vi "Action Worker Mode Example.vi"() -> ()   [LabVIEW 2017, in "Action Worker Mode Example.lvlib"]
doc: "### Caller Program (Action Worker Mode Example.vi)\n\n#### Overview\n\nDemonstrates the Worker Mode within the CSM framework. In this example, four workers run in the background, collectively forming a CSM module in Worker Mode.\n\n#### Introduction\n\nThis example demonstrates the Worker Mode within the CSM framework. In Worker Mode, multiple cloneable CSM instances run as nodes. To avoid naming conflicts, the module name is appended with a \"#\" suffix, informing the CSM framework that this is a worker module. When a message is sent to the workers, the message is handled using a fair queuing mechanism, where the first available worker module processes the message. From an external perspective, the system behaves as if only a single module is running, and all CSM concepts, such as synchronous, asynchronous, and broadcast, remain unchanged.\n\nIn this example, four workers run in the background.\n\n#### Steps\n\n- Step1: Use the Advanced VI to mark the CSM module as Worker Mode (adding `#` as a suffix). If you are familiar with CSM rules, you can also type the correct name suffix directly without using this VI. Then, asynchronously call the 4 worker CSM modules without waiting for a reply. Alternatively, you can call the 4 worker CSM modules synchronously, or even asynchronously with a reply (refer to the code in the Disabled cases).\n- Step2: This loop is the main program module, named `WorkerModeExample`.\n- Step3: Use a While Loop to retrieve status information for all running CSM modules, including names, modes, instance counts, and the number of message queues to be processed. Use the Advanced VI to stop the While Loop. Once the caller/main CSM module exits, the While Loop will stop.\n- Step4:\n - Step4.1: UI Event Handling. After the user clicks any of the following six user buttons, an inter-module message is sent to the first available worker CSM module.\n - \"DoSth: DoA -> Worker\"\n - \"DoSth: DoA -@ Worker\"\n - \"DoSth: Error -> Worker\"\n - \"DoSth: Error -@ Worker\"\n - \"Macro: Exit -@ Worker\"\n - \"Macro: Exit -> Worker\"\n - Step4.2: Add a Response Source Manager indicator to the UI to handle \"Async Response\" and \"Response\" cases.\n- Step5: Module Exit. In the `Macro: Exit` message, use the CSM - Build Exit Messages of CSMs VI to create synchronous `Macro: Exit` messages for all running CSM worker modules. You can also manually type the inter-module messages, but be aware of how many worker modules are running. One message is required for each running worker instance. Then, send the local message `Macro: Exit` to the caller/main CSM module. All CSM modules will then exit sequentially."
uses:
  Action Worker Mode Example.lvlib
  user.lib/_NEVSTOP/Communicable State Machine(CSM)/_Support/Typedef/_CSM_Response Source Message.ctl
  user.lib/_NEVSTOP/Communicable State Machine(CSM)/_Support/Typedef/_CSM_MODE.ctl
  user.lib/_NEVSTOP/Communicable State Machine(CSM)/AdvanceAPI/CSM - Make String Arguments Safe.vi
  user.lib/_NEVSTOP/Communicable State Machine(CSM)/AdvanceAPI/CSM - Break Down Multiple States String.vi
  user.lib/_NEVSTOP/Communicable State Machine(CSM)/AdvanceAPI/CSM - Compact Multiple States.vi
  user.lib/_NEVSTOP/Communicable State Machine(CSM)/AdvanceAPI/CSM - Keywords.vi
  user.lib/_NEVSTOP/Communicable State Machine(CSM)/Communicable State Machine.lvlib
panel:
  in  "All?":bool
  out "Module List":T2(array[cluster])
  out ">> Response Source Message >>":T3
  in  "DoSth: Error -> Worker":bool
  in  "DoSth: Error -@ Worker":bool
  in  "Macro: Exit -> Worker":bool
  in  "Macro: Exit -@ Worker":bool
  in  "DoSth: DoA -@ Worker":bool
  out "State History":string
  in  "DoSth: DoA -> Worker":bool
  # "#CSM-Example Overview\n\nDemonstrates the Worker Mode within the CSM framework. In this example, four workers run in the background, collectively forming a CSM module in Worker Mode."
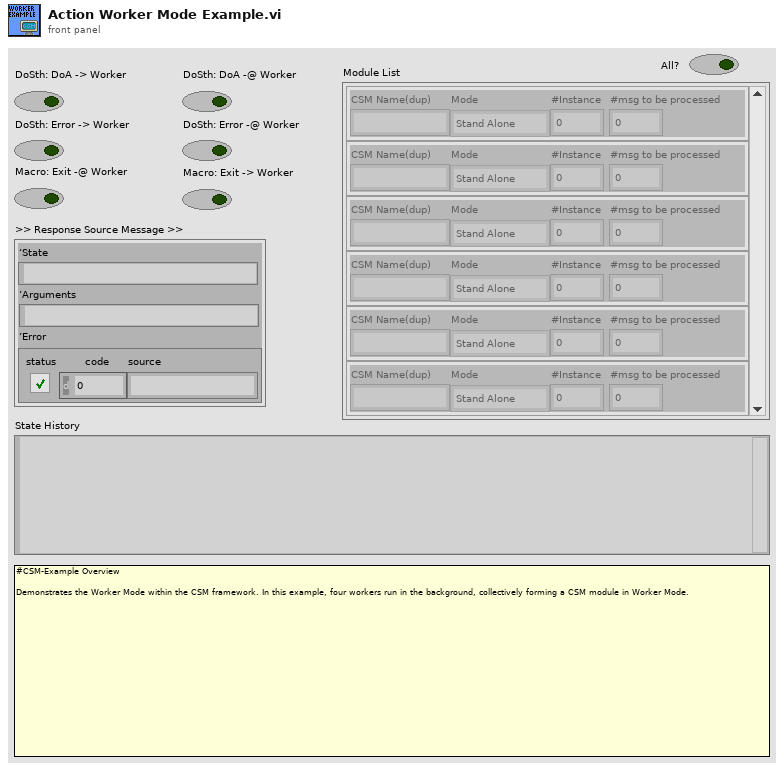
[diagram p1: front panel]
types:
  T1 = typedef "Communicable State Machine.lvlib/_CSM_MODE.ctl" = enum16{"Not Exist", "Stand Alone", "CSM", "Worker", "Worker Agent", "Chain Node", "Chain"}
  T2 = cluster{"CSM Name(dup)":string, "Mode":T1, "#Instance":i32, "#msg to be processed":i32}[]
  T3 = typedef "Communicable State Machine.lvlib/_CSM_Response Source Message.ctl" = cluster{"‘State":string, "’Arguments":string, "’Error":errorcluster}
  T4 = enum32{"Invalid", "Standard", "Closed", "Hidden", "Minimized", "Maximized"}
  T5 = enum32{"invalid app kind", "Development System", "Run Time System", "Student Edition", "Embedded LabVIEW", "Evaluation", "Custom"}
  T6 = cluster{"Current VI Reference":refnum<vi>, "Close Panel on Exit?":bool}
  T7 = cluster{"Core":cluster{"Current VI Reference":refnum<vi>, "Close Panel on Exit?":bool}, "Your Boolean data":bool, "Your string data":string}
  T8 = cluster{"CSM Name (Dup)":string, "Mode":T1, "#Nodes":i32, "#Elements In Queue":i32}
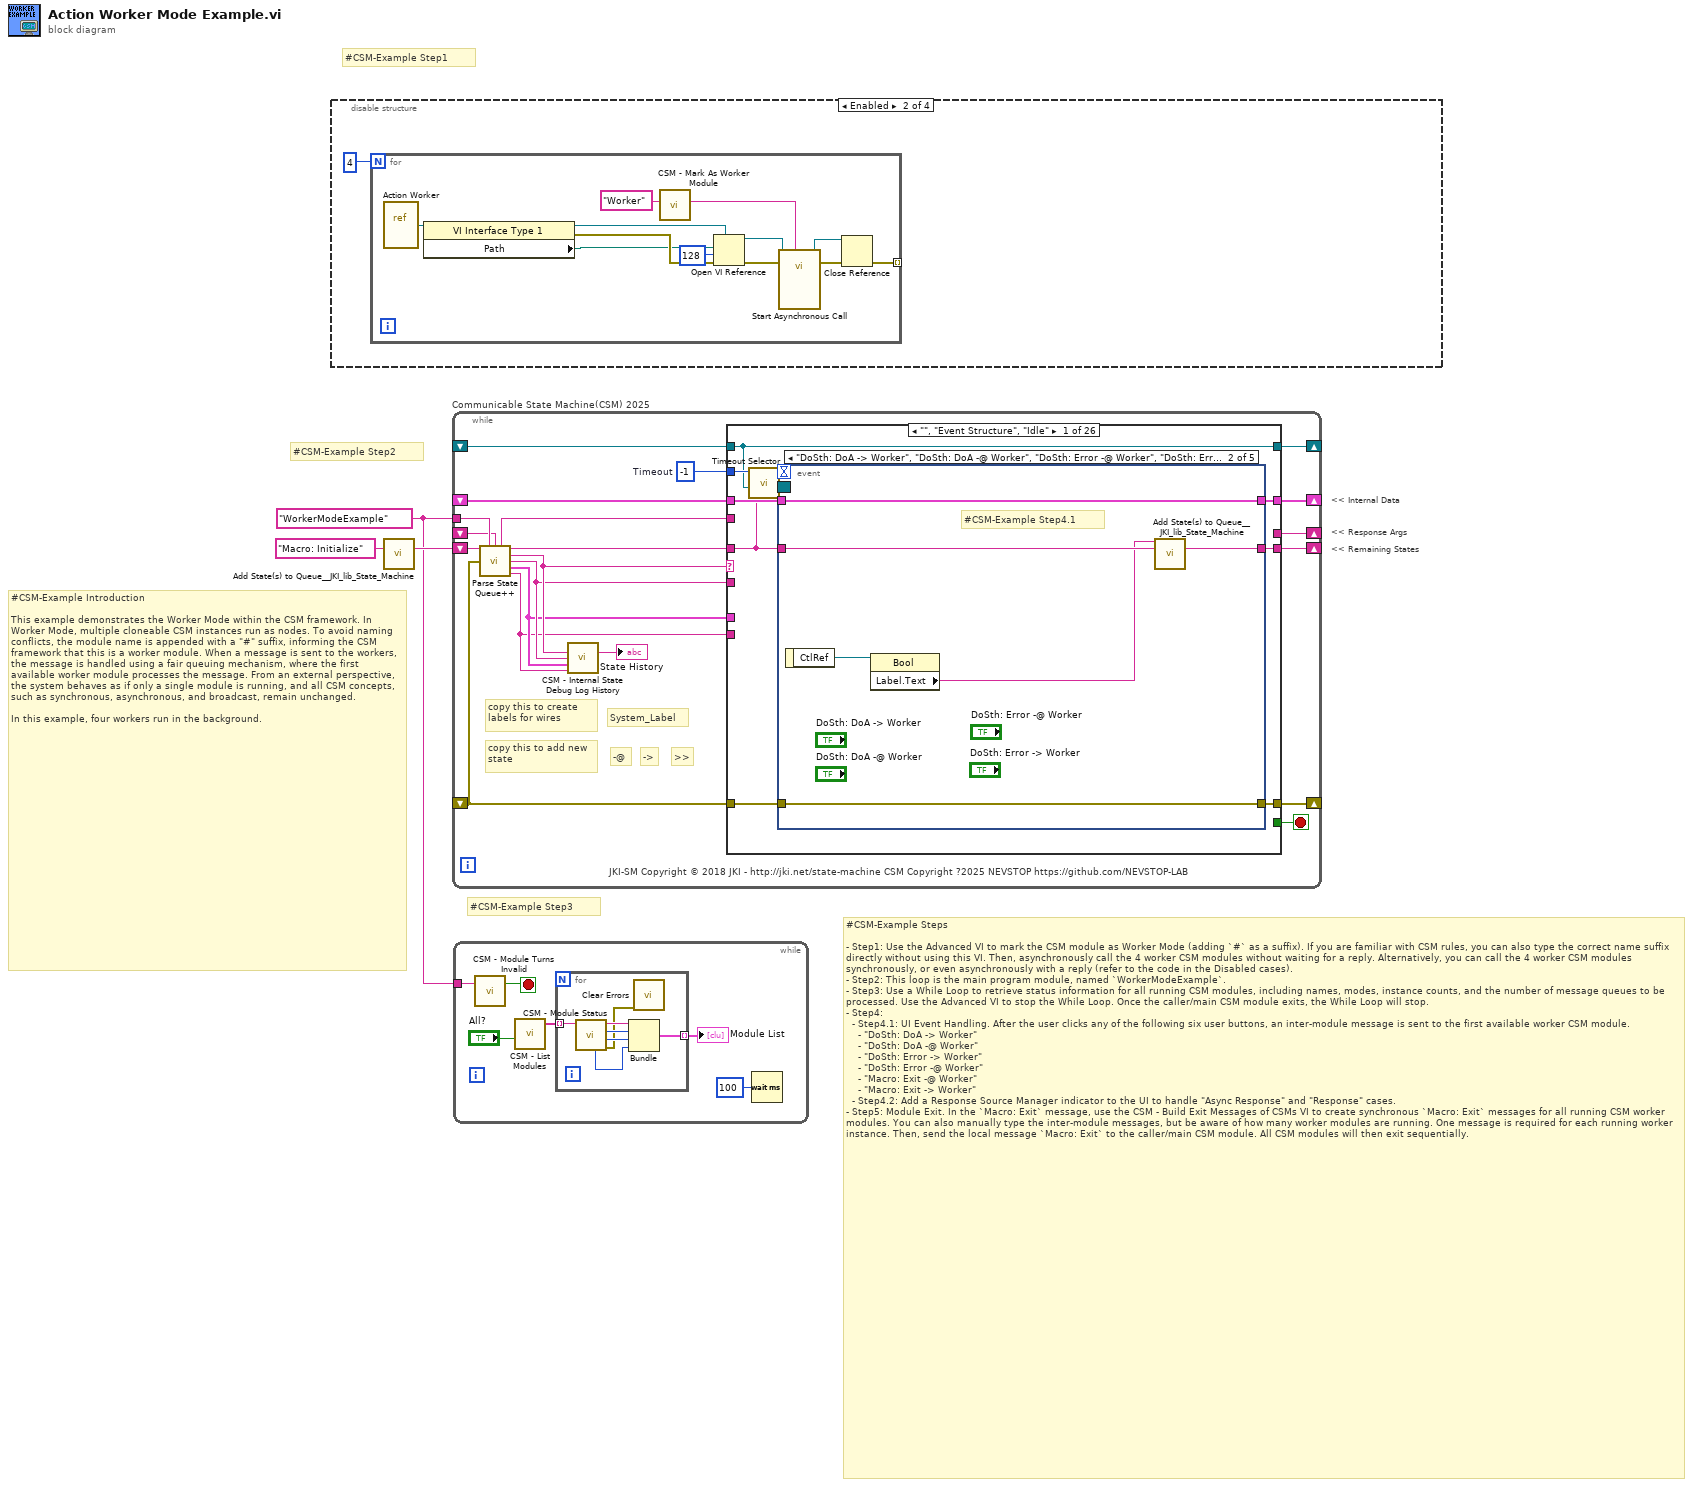
[diagram p0: block diagram]
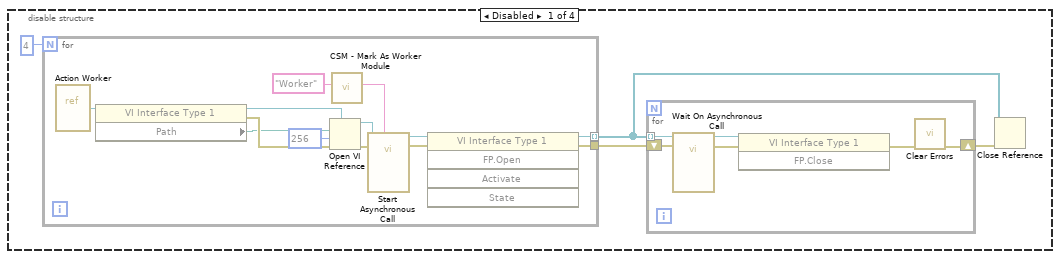
[diagram p2: hidden frame]
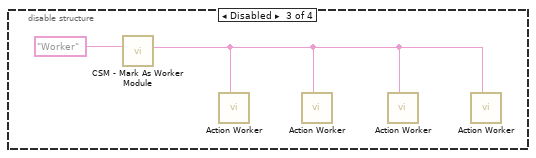
[diagram p3: hidden frame]
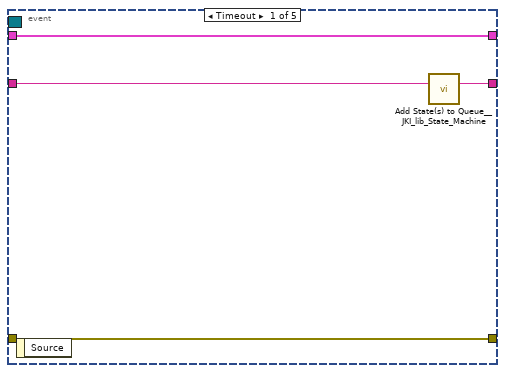
[diagram p5: hidden frame]
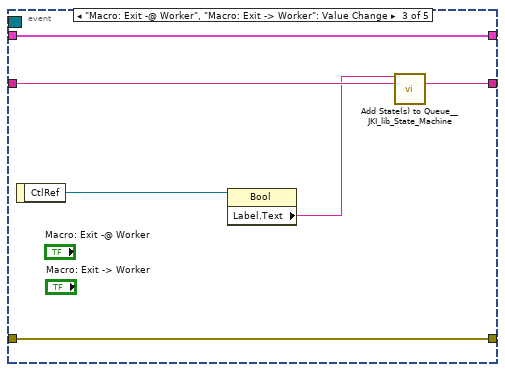
[diagram p6: hidden frame]
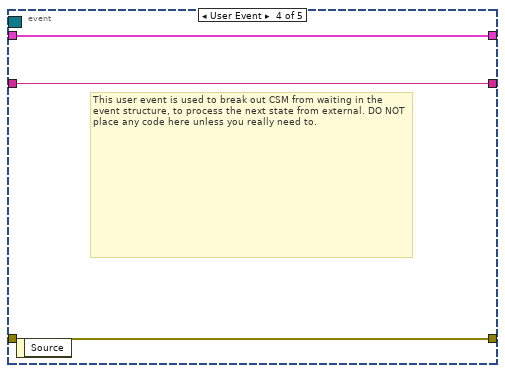
[diagram p7: hidden frame]
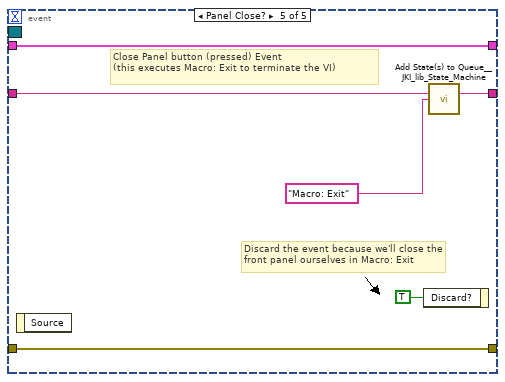
[diagram p8: hidden frame]
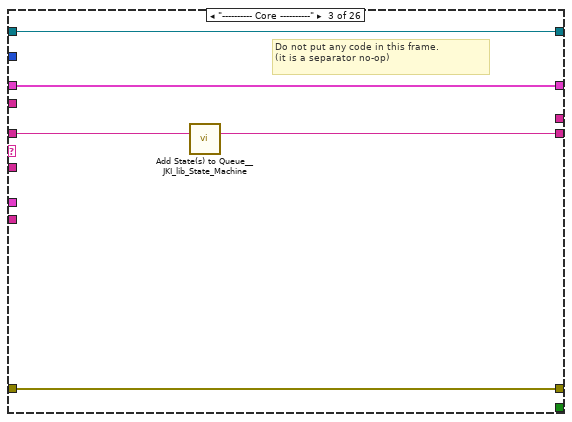
[diagram p10: hidden frame]
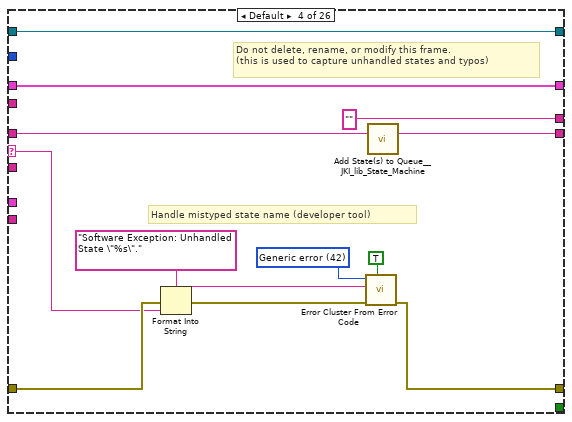
[diagram p11: hidden frame]
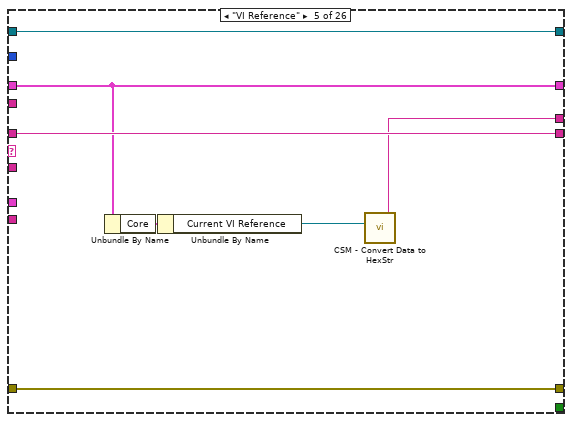
[diagram p12: hidden frame]
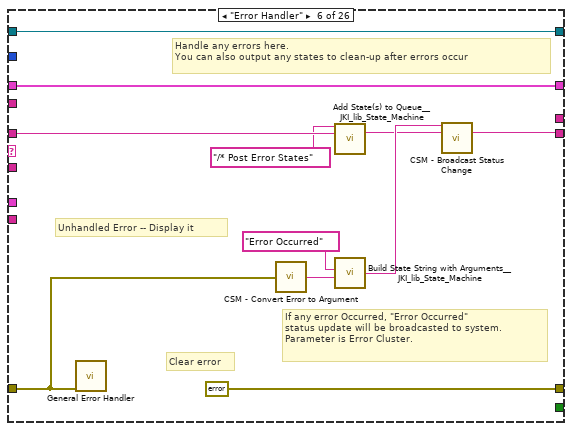
[diagram p13: hidden frame]
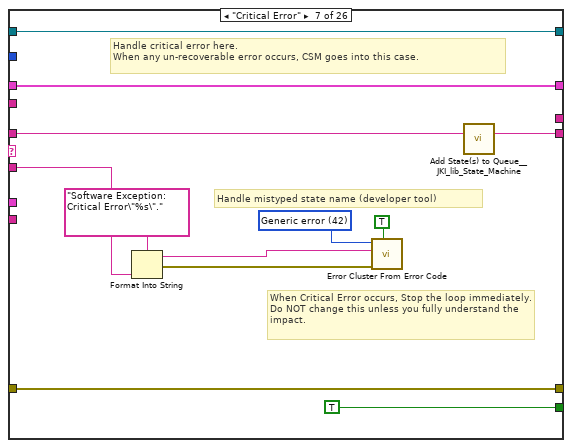
[diagram p14: hidden frame]
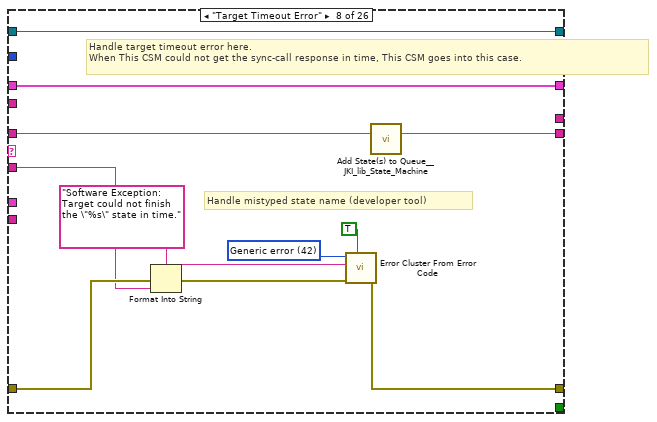
[diagram p15: hidden frame]
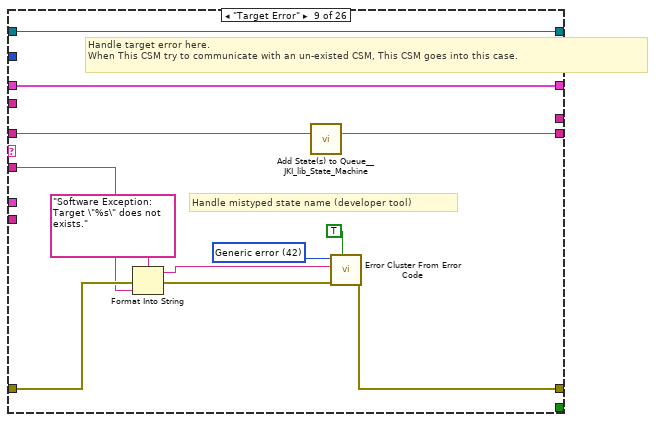
[diagram p16: hidden frame]
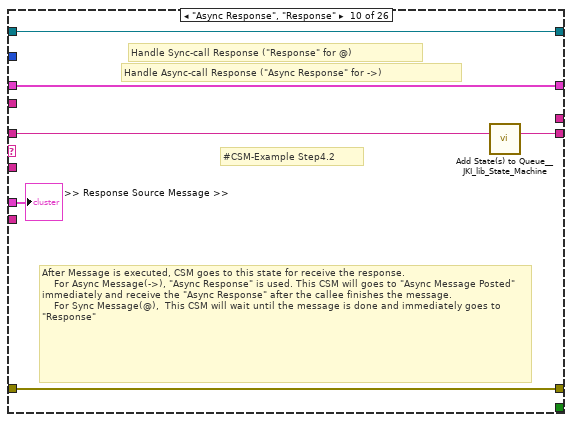
[diagram p17: hidden frame]
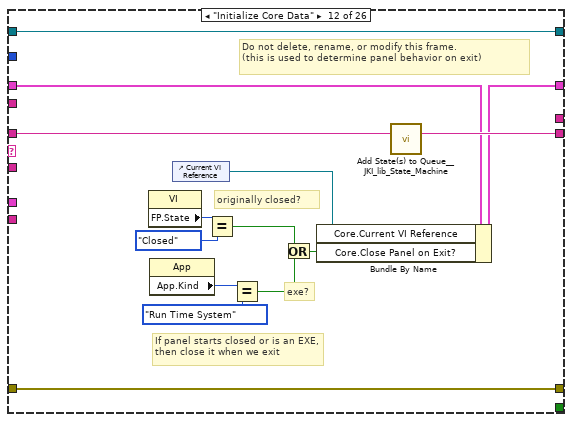
[diagram p19: hidden frame]
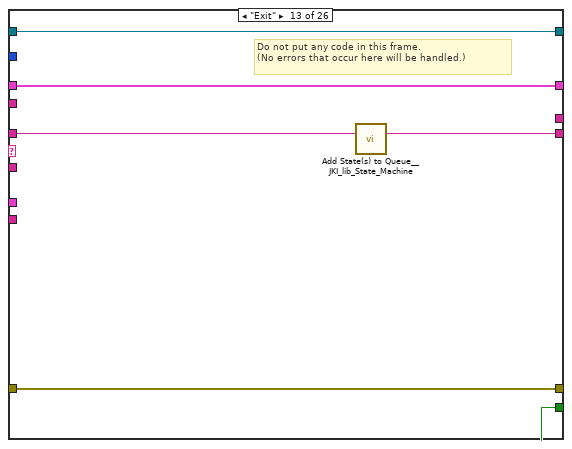
[diagram p20: hidden frame]
diagram:
  w1 = "WorkerModeExample" ("Name (\"\" to Use UUID)")
  # "#CSM-Example Step1"
  # "#CSM-Example Step3"
  # "#CSM-Example Step2"
  # "#CSM-Example Steps\n\n- Step1: Use the Advanced VI to mark the CSM module as Worker Mode (adding `#` as a suffix). If you are familiar with CSM rules, you can also type the correct name suffix directly without using this VI. Then, asynchronously call the 4 worker CSM modules without waiting for a reply. Alternatively, you can call the 4 worker CSM modules synchronously, or even asynchronously with a reply (refer to the code in the Disabled cases).\n- Step2: This loop is the main program module, named `WorkerModeExample`.\n- Step3: Use a While Loop to retrieve status information for all running CSM modules, including names, modes, instance counts, and the number of message queues to be processed. Use the Advanced VI to stop the While Loop. Once the caller/main CSM module exits, the While Loop will stop.\n- Step4:\n  - Step4.1: UI Event Handling. After the user clicks any of the following six user buttons, an inter-module message is sent to the first available worker CSM module.\n    - \"DoSth: DoA -> Worker\"\n    - \"DoSth: DoA -@ Worker\"\n    - \"DoSth: Error -> Worker\"\n    - \"DoSth: Error -@ Worker\"\n    - \"Macro: Exit -@ Worker\"\n    - \"Macro: Exit -> Worker\"\n  - Step4.2: Add a Response Source Manager indicator to the UI to handle \"Async Response\" and \"Response\" cases.\n- Step5: Module Exit. In the `Macro: Exit` message, use the CSM - Build Exit Messages of CSMs VI to create synchronous `Macro: Exit` messages for all running CSM worker modules. You can also manually type the inter-module messages, but be aware of how many worker modules are running. One message is required for each running worker instance. Then, send the local message `Macro: Exit` to the caller/main CSM module. All CSM modules will then exit sequentially."
  # "#CSM-Example Introduction\n\nThis example demonstrates the Worker Mode within the CSM framework. In Worker Mode, multiple cloneable CSM instances run as nodes. To avoid naming conflicts, the module name is appended with a \"#\" suffix, informing the CSM framework that this is a worker module. When a message is sent to the workers, the message is handled using a fair queuing mechanism, where the first available worker module processes the message. From an external perspective, the system behaves as if only a single module is running, and all CSM concepts, such as synchronous, asynchronous, and broadcast, remain unchanged.\n\nIn this example, four workers run in the background."
  # "<< Internal Data"
  # "<< Response Args"
  # "<< Remaining States"
  n1 = disable-structure shown="Enabled" {
    frame Disabled {
      n2 = for {
        N: 4 -> [_]
        tunnel: [w17] -> w4
        tunnel: [w18] -> w5 mode=indexing
        n3 = vi-ref "Action Worker.vi"() -> (w21:refnum<vi>)
        n4 = property class="VI Interface Type 1"(reference=w21) -> (reference out=w25:refnum<vi>, error out=w23:errorcluster, "Path"=w22:path)  [unwired: 1 in]
        n5 = Open VI Reference(type specifier VI Refnum (for type only)=w25, vi path=w22, options=256, error in (no error)=w23) -> (vi reference=w24:refnum<vi>, error out=w20:errorcluster)  [unwired: 2 in]
        n6 = call "CSM - Mark As Worker Module.vi"("CSM Name"="Worker" ("Name (\"\" to Use UUID)")) -> ("CSM Name (Marked As Worker)"=w14:string)  [unwired: 9 in]
        n7 = call-by-ref "Start Asynchronous Call"(reference=w24, error in=w20, "Name(\"\" to use uuid)"=w14) -> (reference out=w19:refnum<vi>, error out=w16:errorcluster)  [unwired: 11 in]
        n8 = invoke class="VI Interface Type 1" method="FP.Open"(reference=w19, error in=w16) -> (reference out=w18:refnum<vi>, error out=w17:errorcluster)  [unwired: 3 in, 3 out]
      }
      n9 = for {
        shift-right: [w8] -> w7
        shift-left: w4 -> [w13]
        tunnel: w5 -> [w12] mode=indexing
        n10 = call-by-ref "Wait On Asynchronous Call"(reference=w12, error in=w13) -> (reference out=w11:refnum<vi>, error out=w9:errorcluster)  [unwired: 12 in]
        n11 = invoke class="VI Interface Type 1" method="FP.Close"(reference=w11, error in=w9) -> (error out=w10:errorcluster)  [unwired: 1 in, 2 out]
        n12 = call <vilib>:"Clear Errors.vi"("error in (no error)"=w10) -> ("error out"=w8:errorcluster)  [unwired: 5 in, 1 out]
      }
      n13 = Close Reference(reference=w5, error in (no error)=w7) -> ()  [unwired: 1 out]
    }
    frame Enabled {
      n14 = for {
        N: 4 -> [_]
        tunnel: [w30] -> _ mode=indexing
        n15 = vi-ref "Action Worker.vi"() -> (w35:refnum<vi>)
        n16 = property class="VI Interface Type 1"(reference=w35) -> (reference out=w38:refnum<vi>, error out=w37:errorcluster, "Path"=w36:path)  [unwired: 1 in]
        n17 = call "CSM - Mark As Worker Module.vi"("CSM Name"="Worker" ("Name (\"\" to Use UUID)")) -> ("CSM Name (Marked As Worker)"=w33:string)  [unwired: 9 in]
        n18 = Open VI Reference(type specifier VI Refnum (for type only)=w38, vi path=w36, options=128, error in (no error)=w37) -> (vi reference=w29:refnum<vi>, error out=w28:errorcluster)  [unwired: 2 in]
        n19 = call-by-ref "Start Asynchronous Call"(reference=w29, error in=w28, "Name(\"\" to use uuid)"=w33) -> (reference out=w31:refnum<vi>, error out=w32:errorcluster)  [unwired: 11 in]
        n20 = Close Reference(reference=w31, error in (no error)=w32) -> (error out=w30:errorcluster)
      }
    }
    frame Disabled {
      n21 = call "CSM - Mark As Worker Module.vi"("CSM Name"="Worker" ("Name (\"\" to Use UUID)")) -> ("CSM Name (Marked As Worker)"=w40:string)  [unwired: 9 in]
      n22 = call "Action Worker.vi"("Name (\"\" to Use UUID)"=w40) -> ()  [unwired: 11 in]
      n23 = call "Action Worker.vi"("Name (\"\" to Use UUID)"=w40) -> ()  [unwired: 11 in]
      n24 = call "Action Worker.vi"("Name (\"\" to Use UUID)"=w40) -> ()  [unwired: 11 in]
      n25 = call "Action Worker.vi"("Name (\"\" to Use UUID)"=w40) -> ()  [unwired: 11 in]
    }
    frame Disabled {
    }
  }
  n26 = call <vilib>:"Add State(s) to Queue__JKI_lib_State_Machine.vi"("State(s) in (\"\")"="Macro: Initialize") -> ("States Out"=w3:string)  [unwired: 14 in]
  n27 = while "Communicable State Machine(CSM) 2025" {
    shift-right: [w56] -> _
    shift-left: _ -> [w55]
    shift-right: [w59] -> _
    shift-left: _ -> [w53]
    shift-right: [w58] -> _
    shift-left: w3 -> [w60]
    tunnel: w1 -> [w49]
    shift-right: [w52] -> _
    shift-left: _ -> [w43]
    shift-right: [w51] -> _
    shift-left: _ -> [w50]
    stop <- w57 stop-if-true
    w54 = -1  # Timeout
    # "JKI-SM Copyright © 2018 JKI - http://jki.net/state-machine CSM Copyright ?2025 NEVSTOP https://github.com/NEVSTOP-LAB"
    # "copy this to add new state"
    # ">>"
    # "->"
    # "-@"
    # "copy this to create labels for wires"
    # "System_Label"
    n28 = call "Parse State Queue++.vi"("State Queue"=w60, "Name (\"\" to Use UUID)"=w49, "Response Arguments"=w43, "Previous Error"=w53) -> ("Name Used"=w44:string, "Remaining States"=w61:string, "Current State"=w48:string, "Arguments"=w47:string, "Additional Information"=w46:T3, "Source CSM"=w45:string)  [unwired: 6 in]
    n29 = call "CSM - Internal State Debug Log History.vi"("State"=w48, "Arguments (\"\")"=w47, ">> Response Source Message >>"=w46, "Source (\"\")"=w45) -> ("Debug Log"=→"State History":string)  [unwired: 11 in]
    n30 = case shown="\"\", \"Event Structure\", \"Idle\"" w48 {
      selector: w48 -> [_ _ _ w107 _ _ _ _ _ _ _ _ _ _ _ _ _ _ _ _ _ _ _ _ _ _]
      tunnel: w61 -> [w62 w98 w104 w111 w123 w135 w145 w153 w165 w174 w180 w195 w201 w206 w214 w221 w226 w232 w236 w242 w247 w254 w270 w340 w346 w359]
      tunnel: w47 -> [_ _ _ _ _ _ w138 w149 w161 _ _ _ _ _ _ _ _ _ _ _ _ w249 w264 _ _ _]
      tunnel: w55 -> [w69 w97 w101 w109 w122 w133 w146 w151 w163 w176 w179 w188 w199 w203 _ w216 w223 w231 w235 w239 w245 w252 w266 w337 w343 w356]
      tunnel: [w68 w99 w102 w113 w124 errorcluster {"status"=FALSE, "code"=0, "source"=""} ("error out") w147 w155 w167 w177 w181 w192 w198 w204 w211 w217 w224 w227 w234 w240 w244 w250 w267 w338 w344 w357] -> w59
      tunnel: w53 -> [w67 w99 w102 w112 w124 w125 w147 w154 w166 w177 w181 w192 w198 w204 w211 w218 w224 _ w237 w240 w244 w251 w268 w338 w344 w357]
      tunnel: [w70 w98 w103 w110 w123 w126 w144 w152 w164 w173 w180 w194 w200 w205 w213 w220 w225 w232 w236 w241 w246 w253 w269 w339 w345 w358] -> w58
      tunnel: [_ _ _ _ _ _ TRUE _ _ _ _ _ TRUE _ _ _ _ _ _ _ _ _ _ _ _ _] -> w57
      tunnel: [w66 w97 w101 w109 w122 w133 w146 w151 w163 w176 w179 w193 w199 w203 w212 w216 w223 w231 w235 w239 w245 w252 w266 w337 w343 w356] -> w56
      tunnel: w54 -> [w65 _ _ _ _ _ _ _ _ _ _ _ _ _ _ _ _ _ _ _ _ _ _ _ _ _]
      tunnel: w45 -> [_ _ _ _ _ _ _ _ _ _ _ _ _ _ _ _ _ _ _ _ _ _ _ _ _ _]
      tunnel: w46 -> [_ _ _ _ _ _ _ _ _ w172 _ _ _ _ _ _ _ _ _ _ _ _ _ _ _ _]
      tunnel: [_ _ _ "" w118 _ _ _ _ _ _ _ _ _ _ _ _ _ _ _ _ _ _ _ _ _] -> w52
      tunnel: [w64 w96 w100 w105 w121 w131 w136 w148 w160 w175 w178 w182 w196 w202 w207 w215 w222 w230 w233 w238 w243 w248 w263 w336 w341 w349] -> w51
      tunnel: w50 -> [w64 w96 w100 w105 w121 w131 w136 w148 w160 w175 w178 w182 w196 w202 w207 w215 w222 _ w233 w238 w243 w248 w263 w336 w341 w349]
      tunnel: w44 -> [_ _ _ _ _ _ _ _ _ _ _ _ _ _ _ _ _ w229 _ _ _ _ _ _ _ _]
      frame "", "Event Structure", "Idle" {
        n31 = call "Timeout Selector.vi"("Remaining States"=w62, "Timeout Expected"=w65) -> ("Timeout"=w63:i32)  [unwired: 5 in]
        n32 = event shown="[1] \"DoSth: DoA -> Worker\", \"DoSth: DoA -@ Worker\", \"DoSth: Error -@ Worker\", \"DoSth: Error -> Worker\": Value Change" {
          selector: w64 -> [_ _ _ _ _]
          dyn-events: _ -> [_ _ _ _ _]
          timeout: w63 -> [_ _ _ _ _]
          tunnel: w62 -> [w74 w78 w84 w88 w95]
          tunnel: [w73 w77 w83 w88 w94] -> w70
          tunnel: w69 -> [w71 w79 w85 w89 w92]
          tunnel: [w72 w80 w86 w87 w93] -> w68
          tunnel: w67 -> [w72 w80 w86 w87 w93]
          tunnel: [w71 w79 w85 w89 w92] -> w66
          event Timeout {
            n33 = event-data() -> ()  [unwired: 1 in, 1 out]
            n34 = call <vilib>:"Add State(s) to Queue__JKI_lib_State_Machine.vi"("State(s) in (\"\")"=w74) -> ("States Out"=w73:string)  [unwired: 14 in]
          }
          event "DoSth: DoA -> Worker", "DoSth: DoA -@ Worker", "DoSth: Error -@ Worker", "DoSth: Error -> Worker": Value Change {
            # "#CSM-Example Step4.1"
            n35 = event-data() -> ("CtlRef"=w76:refnum<vi>)  [unwired: 1 in]
            n36 = property class="Bool"(reference=w76) -> ("Label.Text"=w75:string)  [unwired: 1 in, 2 out]
            n37 = call <vilib>:"Add State(s) to Queue__JKI_lib_State_Machine.vi"("State(s) in Front (\"\")"=w75, "State(s) in (\"\")"=w78) -> ("States Out"=w77:string)  [unwired: 13 in]
          }
          event "Macro: Exit -@ Worker", "Macro: Exit -> Worker": Value Change {
            n38 = event-data() -> ("CtlRef"=w82:refnum<vi>)  [unwired: 1 in]
            n39 = property class="Bool"(reference=w82) -> ("Label.Text"=w81:string)  [unwired: 1 in, 2 out]
            n40 = call <vilib>:"Add State(s) to Queue__JKI_lib_State_Machine.vi"("State(s) in Front (\"\")"=w81, "State(s) in (\"\")"=w84) -> ("States Out"=w83:string)  [unwired: 13 in]
          }
          event User Event {
            # "This user event is used to break out CSM from waiting in the event structure, to process the next state from external. DO NOT place any code here unless you really need to."
            n41 = event-data() -> ()  [unwired: 1 in, 1 out]
          }
          event Panel Close? {
            # "Discard the event because we'll close the front panel ourselves in Macro: Exit"
            # "Close Panel button (pressed) Event\n(this executes Macro: Exit to terminate the VI)"
            n42 = event-data() -> ()  [unwired: 1 in, 1 out]
            n43 = event-data("Discard?"=TRUE) -> ()  [unwired: 1 in, 1 out]
            n44 = call <vilib>:"Add State(s) to Queue__JKI_lib_State_Machine.vi"("State(s) in (\"\")"=w95, "State(s) at Back (\"\")"="Macro: Exit") -> ("States Out"=w94:string)  [unwired: 13 in]
          }
        }
      }
      frame "CSM Documentation" {
        # "#CSM README FIRST\n\nCSM is a LabVIEW application framework that builds upon JKI State Machine (JKISM). It follows the pattern of JKISM and extends the keywords to describe message communication between CSM modules, including concepts such as Sync-Message, Async-Message, Subscription/Unsubscription of status - essential elements for creating reusable code modules. For more information, please visit the CSM wiki: https://github.com/NEVSTOP-LAB/JKI-State-Machine-Plus-Plus/wiki\n\nFor instructions on JKI State Machine, visit: http://jki.net/state-machine/\nFor information about CSM, visit: https://github.com/NEVSTOP-LAB"
        # "CSM Documentation"
      }
      frame "---------- Core ----------" {
        # "Do not put any code in this frame.\n(it is a separator no-op)"
        n45 = call <vilib>:"Add State(s) to Queue__JKI_lib_State_Machine.vi"("State(s) in (\"\")"=w104) -> ("States Out"=w103:string)  [unwired: 14 in]
      }
      frame Default {
        w116 = 42 items=["No error", "Argument error", "Memory is full", "Out of zone", "End of file", "File already open", "Generic file I/O error", "File not found", "File permission error", "Disk is full", "Duplicate path", "Too many files open", "System feature not enabled", "Resource file not found", "Cannot add resource", "Resource not found", "Image not found", "Image memory error", "Pen does not exist", "Config type invalid", "Config token not found", "Config parse error", "Config memory error", "Bad external code format", "Bad external code offset", "External code not present", "Null window", "Destroy window error", "Null menu", "Print aborted", "Bad print record", "Print driver error", "Windows error during printing", "Memory error during printing", "Print dialog error", "Generic print error", "Invalid device refnum", "Device not found", "Device parameter error", "Device unit error", "Cannot open device", "Device call aborted", "Generic error", "Cancelled by user", "Object ID too low", "Object ID too high", "Object not in heap", "Unknown heap", "Unknown object (invalid DefProc)", "Unknown object (DefProc not in table)", "Message out of range", "Invalid (null) method", "Unknown message", "Manager call not supported", "Bad address", "Network operation in progress", "Network operation timed out", "Connection is busy", "Network attribute not supported", "Network error", "Address in use", "System out of memory", "Connection aborted", "Connection refused", "Not connected", "Already connected", "Connection closed", "Initialization error (interapplication manager)", "Bad occurrence", "Wait on unbound occurrence handler", "Occurrence queue overflow", "Datalog type conflict", "Unused", "Unrecognized type (interapplication manager)", "Memory corrupt", "Failed to make temporary DLL", "Old CIN version", "Drag socket not found", "Failed to load drop-object", "Failed to register OLE object", "Failed to release OLE object", "Format specifier type mismatch", "Unknown format specifier", "Too few format specifiers", "Too many format specifiers", "Scan failed", "Newer CIN version", "Error converting to variant", "Runtime menu error", "Password tampered", "Variant attribute not found", "Incompatible variant data type", "Event data is not available", "Event Store is not present", "Occurrence is not found", "Event Queue is not created", "Event info is not available", "Refnum passed is NULL", "Error retrieving Class GUID", "Error retrieving CoClass GUID", "Error retrieving TypeLib GUID.", "Bad built application magic bytes.", "Specific driver is different from the specific driver associated with the Logical Name.", "There is no session opened to the class driver.", "Max Error", "MAX - Error with config objects", "MAX - Error loading configuration", "MAX - Group not supported"]
        # "Do not delete, rename, or modify this frame.\n(this is used to capture unhandled states and typos)"
        # "Handle mistyped state name (developer tool)"
        n46 = Format Into String(format string="Software Exception: Unhandled State \"%s\"." ("message"), error in=w112, w107) -> (resulting string=w115:string, error out=w114:errorcluster)  [unwired: 1 in]
        n47 = call <vilib>:"Error Cluster From Error Code.vi"("show call chain? (False)"=TRUE, "error in (no error)"=w114, "error message (\"\")"=w115, "error code (0)"=w116) -> ("error out"=w113:errorcluster)  [unwired: 5 in]
        n48 = call <vilib>:"Add State(s) to Queue__JKI_lib_State_Machine.vi"("State(s) in (\"\")"=w111) -> ("States Out"=w110:string)  [unwired: 14 in]
      }
      frame "VI Reference" {
        n49 = Unbundle By Name(w122) -> ("Core"=w120:T6)
        n50 = Unbundle By Name(w120) -> ("Current VI Reference"=w119:refnum<vi>)
        n51 = call "CSM - Convert Data to HexStr.vi"("Variant"=w119) -> ("HEX String (0-9,A-F)"=w118:string)  [unwired: 8 in]
      }
      frame "Error Handler" {
        # "If any error Occurred, \"Error Occurred\" \nstatus update will be broadcasted to system.\nParameter is Error Cluster."
        # "Unhandled Error -- Display it"
        # "Handle any errors here.\nYou can also output any states to clean-up after errors occur"
        # "Clear error"
        n52 = call <vilib>:"General Error Handler.vi"("error in (no error)"=w125) -> ()  [unwired: 10 in, 5 out]
        n53 = call "CSM - Convert Error to Argument.vi"("Error"=w125) -> ("Argument"=w129:string)  [unwired: 4 in]
        n54 = call <vilib>:"Add State(s) to Queue__JKI_lib_State_Machine.vi"("State(s) in Front (\"\")"="/* Post Error States", "State(s) in (\"\")"=w135) -> ("States Out"=w127:string)  [unwired: 13 in]
        n55 = call <vilib>:"Build State String with Arguments__JKI_lib_State_Machine.vi"("Arguments (\"\")"=w129, "State"="Error Occurred" ("Status with Arguments")) -> ("State with Arguments"=w128:string)  [unwired: 4 in]
        n56 = call "CSM - Broadcast Status Change.vi"("Status With Arguments"=w128, "State Queue"=w127) -> ("Remaining States"=w126:string)  [unwired: 13 in]
      }
      frame "Critical Error" {
        w142 = 42 items=["No error", "Argument error", "Memory is full", "Out of zone", "End of file", "File already open", "Generic file I/O error", "File not found", "File permission error", "Disk is full", "Duplicate path", "Too many files open", "System feature not enabled", "Resource file not found", "Cannot add resource", "Resource not found", "Image not found", "Image memory error", "Pen does not exist", "Config type invalid", "Config token not found", "Config parse error", "Config memory error", "Bad external code format", "Bad external code offset", "External code not present", "Null window", "Destroy window error", "Null menu", "Print aborted", "Bad print record", "Print driver error", "Windows error during printing", "Memory error during printing", "Print dialog error", "Generic print error", "Invalid device refnum", "Device not found", "Device parameter error", "Device unit error", "Cannot open device", "Device call aborted", "Generic error", "Cancelled by user", "Object ID too low", "Object ID too high", "Object not in heap", "Unknown heap", "Unknown object (invalid DefProc)", "Unknown object (DefProc not in table)", "Message out of range", "Invalid (null) method", "Unknown message", "Manager call not supported", "Bad address", "Network operation in progress", "Network operation timed out", "Connection is busy", "Network attribute not supported", "Network error", "Address in use", "System out of memory", "Connection aborted", "Connection refused", "Not connected", "Already connected", "Connection closed", "Initialization error (interapplication manager)", "Bad occurrence", "Wait on unbound occurrence handler", "Occurrence queue overflow", "Datalog type conflict", "Unused", "Unrecognized type (interapplication manager)", "Memory corrupt", "Failed to make temporary DLL", "Old CIN version", "Drag socket not found", "Failed to load drop-object", "Failed to register OLE object", "Failed to release OLE object", "Format specifier type mismatch", "Unknown format specifier", "Too few format specifiers", "Too many format specifiers", "Scan failed", "Newer CIN version", "Error converting to variant", "Runtime menu error", "Password tampered", "Variant attribute not found", "Incompatible variant data type", "Event data is not available", "Event Store is not present", "Occurrence is not found", "Event Queue is not created", "Event info is not available", "Refnum passed is NULL", "Error retrieving Class GUID", "Error retrieving CoClass GUID", "Error retrieving TypeLib GUID.", "Bad built application magic bytes.", "Specific driver is different from the specific driver associated with the Logical Name.", "There is no session opened to the class driver.", "Max Error", "MAX - Error with config objects", "MAX - Error loading configuration", "MAX - Group not supported"]
        # "Handle critical error here.\nWhen any un-recoverable error occurs, CSM goes into this case."
        # "When Critical Error occurs, Stop the loop immediately. Do NOT change this unless you fully understand the impact."
        # "Handle mistyped state name (developer tool)"
        n57 = Format Into String(format string="Software Exception: Critical Error\"%s\"." ("message"), w138) -> (resulting string=w141:string, error out=w140:errorcluster)  [unwired: 2 in]
        n58 = call <vilib>:"Error Cluster From Error Code.vi"("show call chain? (False)"=TRUE, "error in (no error)"=w140, "error message (\"\")"=w141, "error code (0)"=w142) -> ()  [unwired: 5 in, 1 out]
        n59 = call <vilib>:"Add State(s) to Queue__JKI_lib_State_Machine.vi"("State(s) in (\"\")"=w145) -> ("States Out"=w144:string)  [unwired: 14 in]
      }
      frame "Target Timeout Error" {
        w158 = 42 items=["No error", "Argument error", "Memory is full", "Out of zone", "End of file", "File already open", "Generic file I/O error", "File not found", "File permission error", "Disk is full", "Duplicate path", "Too many files open", "System feature not enabled", "Resource file not found", "Cannot add resource", "Resource not found", "Image not found", "Image memory error", "Pen does not exist", "Config type invalid", "Config token not found", "Config parse error", "Config memory error", "Bad external code format", "Bad external code offset", "External code not present", "Null window", "Destroy window error", "Null menu", "Print aborted", "Bad print record", "Print driver error", "Windows error during printing", "Memory error during printing", "Print dialog error", "Generic print error", "Invalid device refnum", "Device not found", "Device parameter error", "Device unit error", "Cannot open device", "Device call aborted", "Generic error", "Cancelled by user", "Object ID too low", "Object ID too high", "Object not in heap", "Unknown heap", "Unknown object (invalid DefProc)", "Unknown object (DefProc not in table)", "Message out of range", "Invalid (null) method", "Unknown message", "Manager call not supported", "Bad address", "Network operation in progress", "Network operation timed out", "Connection is busy", "Network attribute not supported", "Network error", "Address in use", "System out of memory", "Connection aborted", "Connection refused", "Not connected", "Already connected", "Connection closed", "Initialization error (interapplication manager)", "Bad occurrence", "Wait on unbound occurrence handler", "Occurrence queue overflow", "Datalog type conflict", "Unused", "Unrecognized type (interapplication manager)", "Memory corrupt", "Failed to make temporary DLL", "Old CIN version", "Drag socket not found", "Failed to load drop-object", "Failed to register OLE object", "Failed to release OLE object", "Format specifier type mismatch", "Unknown format specifier", "Too few format specifiers", "Too many format specifiers", "Scan failed", "Newer CIN version", "Error converting to variant", "Runtime menu error", "Password tampered", "Variant attribute not found", "Incompatible variant data type", "Event data is not available", "Event Store is not present", "Occurrence is not found", "Event Queue is not created", "Event info is not available", "Refnum passed is NULL", "Error retrieving Class GUID", "Error retrieving CoClass GUID", "Error retrieving TypeLib GUID.", "Bad built application magic bytes.", "Specific driver is different from the specific driver associated with the Logical Name.", "There is no session opened to the class driver.", "Max Error", "MAX - Error with config objects", "MAX - Error loading configuration", "MAX - Group not supported"]
        # "Handle target timeout error here.\nWhen This CSM could not get the sync-call response in time, This CSM goes into this case."
        # "Handle mistyped state name (developer tool)"
        n60 = Format Into String(format string="Software Exception: Target could not finish the \"%s\" state in time." ("message"), error in=w154, w149) -> (resulting string=w157:string, error out=w156:errorcluster)  [unwired: 1 in]
        n61 = call <vilib>:"Error Cluster From Error Code.vi"("show call chain? (False)"=TRUE, "error in (no error)"=w156, "error message (\"\")"=w157, "error code (0)"=w158) -> ("error out"=w155:errorcluster)  [unwired: 5 in]
        n62 = call <vilib>:"Add State(s) to Queue__JKI_lib_State_Machine.vi"("State(s) in (\"\")"=w153) -> ("States Out"=w152:string)  [unwired: 14 in]
      }
      frame "Target Error" {
        w170 = 42 items=["No error", "Argument error", "Memory is full", "Out of zone", "End of file", "File already open", "Generic file I/O error", "File not found", "File permission error", "Disk is full", "Duplicate path", "Too many files open", "System feature not enabled", "Resource file not found", "Cannot add resource", "Resource not found", "Image not found", "Image memory error", "Pen does not exist", "Config type invalid", "Config token not found", "Config parse error", "Config memory error", "Bad external code format", "Bad external code offset", "External code not present", "Null window", "Destroy window error", "Null menu", "Print aborted", "Bad print record", "Print driver error", "Windows error during printing", "Memory error during printing", "Print dialog error", "Generic print error", "Invalid device refnum", "Device not found", "Device parameter error", "Device unit error", "Cannot open device", "Device call aborted", "Generic error", "Cancelled by user", "Object ID too low", "Object ID too high", "Object not in heap", "Unknown heap", "Unknown object (invalid DefProc)", "Unknown object (DefProc not in table)", "Message out of range", "Invalid (null) method", "Unknown message", "Manager call not supported", "Bad address", "Network operation in progress", "Network operation timed out", "Connection is busy", "Network attribute not supported", "Network error", "Address in use", "System out of memory", "Connection aborted", "Connection refused", "Not connected", "Already connected", "Connection closed", "Initialization error (interapplication manager)", "Bad occurrence", "Wait on unbound occurrence handler", "Occurrence queue overflow", "Datalog type conflict", "Unused", "Unrecognized type (interapplication manager)", "Memory corrupt", "Failed to make temporary DLL", "Old CIN version", "Drag socket not found", "Failed to load drop-object", "Failed to register OLE object", "Failed to release OLE object", "Format specifier type mismatch", "Unknown format specifier", "Too few format specifiers", "Too many format specifiers", "Scan failed", "Newer CIN version", "Error converting to variant", "Runtime menu error", "Password tampered", "Variant attribute not found", "Incompatible variant data type", "Event data is not available", "Event Store is not present", "Occurrence is not found", "Event Queue is not created", "Event info is not available", "Refnum passed is NULL", "Error retrieving Class GUID", "Error retrieving CoClass GUID", "Error retrieving TypeLib GUID.", "Bad built application magic bytes.", "Specific driver is different from the specific driver associated with the Logical Name.", "There is no session opened to the class driver.", "Max Error", "MAX - Error with config objects", "MAX - Error loading configuration", "MAX - Group not supported"]
        # "Handle target error here.\nWhen This CSM try to communicate with an un-existed CSM, This CSM goes into this case."
        # "Handle mistyped state name (developer tool)"
        n63 = Format Into String(format string="Software Exception: Target \"%s\" does not exists." ("message"), error in=w166, w161) -> (resulting string=w169:string, error out=w168:errorcluster)  [unwired: 1 in]
        n64 = call <vilib>:"Add State(s) to Queue__JKI_lib_State_Machine.vi"("State(s) in (\"\")"=w165) -> ("States Out"=w164:string)  [unwired: 14 in]
        n65 = call <vilib>:"Error Cluster From Error Code.vi"("show call chain? (False)"=TRUE, "error in (no error)"=w168, "error message (\"\")"=w169, "error code (0)"=w170) -> ("error out"=w167:errorcluster)  [unwired: 5 in]
      }
      frame "Async Response", "Response" {
        # "#CSM-Example Step4.2"
        # "Handle Async-call Response (\"Async Response\" for ->)"
        # "Handle Sync-call Response (\"Response\" for @)"
        # "After Message is executed, CSM goes to this state for receive the response. \n    For Async Message(->), \"Async Response\" is used. This CSM will goes to \"Async Message Posted\" immediately and receive the \"Async Response\" after the callee finishes the message.\n    For Sync Message(@),  This CSM will wait until the message is done and immediately goes to \"Response\""
        n66 = call <vilib>:"Add State(s) to Queue__JKI_lib_State_Machine.vi"("State(s) in (\"\")"=w174) -> ("States Out"=w173:string)  [unwired: 14 in]
        ">> Response Source Message >>" <- w172
      }
      frame "Async Message Posted" {
        # "Handle post action for async message (->)."
        # "After Async Message is posted (->), CSM goes to this state for post-action. You can use Argument - State to tell which Async Message is called."
      }
      frame "Initialize Core Data" {
        # "Do not delete, rename, or modify this frame.\n(this is used to determine panel behavior on exit)"
        # "originally closed?"
        # "exe?"
        # "If panel starts closed or is an EXE, then close it when we exit"
        n67 = property class="VI"() -> ("FP.State"=w185:T4)  [unwired: 2 in, 2 out]
        n68 = property class="App"() -> ("App.Kind"=w191:T5)  [unwired: 2 in, 2 out]
        n69 = control-ref of="Current VI Reference"() -> (w186:refnum<vi>)
        n70 = Equal?(x=w185, y=T4."Closed" ("Front Panel Window:State")) -> (x = y?=w183:bool)
        n71 = Equal?(x=w191, y=T5."Run Time System" ("Application:Kind")) -> (x = y?=w189:bool)
        n72 = Or(x=w183, y=w189) -> (x .or. y?=w187:bool)
        n73 = Bundle By Name(cluster=w188, "Core.Current VI Reference"=w186, "Core.Close Panel on Exit?"=w187) -> (w193:T7)
        n74 = call <vilib>:"Add State(s) to Queue__JKI_lib_State_Machine.vi"("State(s) in (\"\")"=w195) -> ("States Out"=w194:string)  [unwired: 14 in]
      }
      frame "Exit" {
        # "Do not put any code in this frame.\n(No errors that occur here will be handled.)"
        n75 = call <vilib>:"Add State(s) to Queue__JKI_lib_State_Machine.vi"("State(s) in (\"\")"=w201) -> ("States Out"=w200:string)  [unwired: 14 in]
      }
      frame "---------- Data ----------" {
        # "Do not put any code in this frame.\n(It is a separator no-op. You can make a copy of this frame to create a new Data frame)"
        n76 = call <vilib>:"Add State(s) to Queue__JKI_lib_State_Machine.vi"("State(s) in (\"\")"=w206) -> ("States Out"=w205:string)  [unwired: 14 in]
      }
      frame "Data: Initialize" {
        w208 = T6 {"Current VI Reference"=refnum, "Close Panel on Exit?"=FALSE}  # Core
        w210 = TRUE  # Your Boolean data
        w209 = ""  # Your string data
        # "do not delete - used by framework"
        # "Expand Bundle to add new data elements to shift register data."
        # "Add new data here."
        # "Initialize the shift-register data, here.\n(data names are defined by what you wire into the bundle function)"
        n77 = Bundle("Core"=w208, "Your Boolean data"=w210, "Your string data"=w209) -> (w212:T7)  [unwired: 1 in]
        n78 = call <vilib>:"Add State(s) to Queue__JKI_lib_State_Machine.vi"("State(s) in (\"\")"=w214) -> ("States Out"=w213:string)  [unwired: 14 in]
      }
      frame "Data: Cleanup" {
        # "Cleanup any data and references, here.\n(this is called automatically, by the Macro: Exit)"
        n79 = Unbundle By Name(w216) -> ("Core.Current VI Reference"=w219:refnum<vi>)
        n80 = Close Reference(reference=w219, error in (no error)=w218) -> (error out=w217:errorcluster)
        n81 = call <vilib>:"Add State(s) to Queue__JKI_lib_State_Machine.vi"("State(s) in (\"\")"=w221) -> ("States Out"=w220:string)  [unwired: 14 in]
      }
      frame "---------- Events ----------" {
        # "Do not put any code in this frame.\n(It is a separator no-op. You can make a copy of this frame to create a new UI frame)"
        n82 = call <vilib>:"Add State(s) to Queue__JKI_lib_State_Machine.vi"("State(s) in (\"\")"=w226) -> ("States Out"=w225:string)  [unwired: 14 in]
      }
      frame "Events: Register" {
        # "Register message event to break Waiting in Event structure."
        n83 = call "CSM - Get New State Notifier Event.vi"("Name (\"\" to Use UUID)"=w229) -> ("error out"=w227:errorcluster, "New State Notifier Event"=w228:refnum<user-event>)  [unwired: 9 in]
        n84 = register-events(w228) -> (reference out=w230:refnum<event-registration>)  [unwired: 2 in, 1 out]
      }
      frame "Events: Unregister" {
        n85 = Unregister For Events(event registration refnum=w233, error in=w237) -> (error out=w234:errorcluster)
      }
      frame "---------- UI ----------" {
        # "Do not put any code in this frame.\n(It is a separator no-op. You can make a copy of this frame to create a new UI frame)"
        n86 = call <vilib>:"Add State(s) to Queue__JKI_lib_State_Machine.vi"("State(s) in (\"\")"=w242) -> ("States Out"=w241:string)  [unwired: 14 in]
      }
      frame "UI: Initialize" {
        # "Initialize the User Interface, here.\n(this is called automatically, by the Macro: Init)"
        n87 = call <vilib>:"Add State(s) to Queue__JKI_lib_State_Machine.vi"("State(s) in (\"\")"=w247) -> ("States Out"=w246:string)  [unwired: 14 in]
      }
      frame "UI: Cursor Set" {
        # "Argument"
        # "Set and Unset Cursor Busy.\n(Usage: \"UI: Cursor Set >> Busy|Idle\")"
        n88 = disable-structure shown="Default" {
          disable-tunnel: w251 -> [w257 w262]
          disable-tunnel: [w256 w262] -> w250
          disable-tunnel: w249 -> [w255 _]
          frame condition #0 (active) {
            n89 = case shown="\"Idle\", Default" w255 {
              tunnel: w257 -> [w259 w261]
              tunnel: [w258 w260] -> w256
              frame "Idle", Default {
                n90 = call <vilib>:"Unset Busy.vi"("error in (no error)"=w259) -> ("error out"=w258:errorcluster)  [unwired: 10 in]
              }
              frame "Busy" {
                n91 = call <vilib>:"Set Busy.vi"("error in (no error)"=w261) -> ("error out"=w260:errorcluster)  [unwired: 9 in, 1 out]
              }
            }
          }
          frame condition #1 {
          }
        }
        n92 = call <vilib>:"Add State(s) to Queue__JKI_lib_State_Machine.vi"("State(s) in (\"\")"=w254) -> ("States Out"=w253:string)  [unwired: 14 in]
      }
      frame "UI: Front Panel State" {
        # "Argument"
        # "Set Front Panel Open or Closed\n(Usage: \"UI: Front Panel State >> Open|Close\")"
        n93 = Unbundle By Name(w266) -> ("Core.Current VI Reference"=w265:refnum<vi>)
        n94 = call <vilib>:"Add State(s) to Queue__JKI_lib_State_Machine.vi"("State(s) in (\"\")"=w270) -> ("States Out"=w269:string)  [unwired: 14 in]
        n95 = case shown="\"Minimize\", \"Minimized\"" w264 {
          tunnel: w268 -> [w276 w291 w302 w315 w328]
          tunnel: [w278 w292 w304 w317 w330] -> w267
          tunnel: w265 -> [w277 w289 w303 w316 w329]
          frame "Open", "Standard", Default {
            w271 = T4."Standard" ("State")
            n96 = property class="VI"(reference=w277, error in=w276) -> (reference out=w274:refnum<vi>, error out=w275:errorcluster, "FP.State"=w273:T4)
            n97 = Not Equal?(x=w273, y=w271) -> (x != y?=w272:bool)
            n98 = case shown="True" w272 {
              tunnel: [w282 w284] -> w278
              tunnel: w275 -> [w281 w284]
              tunnel: w274 -> [w280 _]
              tunnel: w271 -> [w279 _]
              frame True {
                n99 = invoke class="VI" method="FP.Open"(reference=w280, error in=w281, "Activate"=TRUE, "State"=w279) -> (error out=w282:errorcluster)  [unwired: 1 in, 4 out]
              }
              frame False {
              }
            }
          }
          frame "Close", "Closed" {
            n100 = property class="VI"(reference=w289, error in=w291) -> (reference out=w288:refnum<vi>, error out=w290:errorcluster, "FP.State"=w286:T4)
            n101 = Not Equal?(x=w286, y=T4."Closed" ("Front Panel Window:State")) -> (x != y?=w285:bool)
            n102 = case shown="True" w285 {
              tunnel: [w293 w296] -> w292
              tunnel: w290 -> [w293 w295]
              tunnel: w288 -> [_ w294]
              frame False {
              }
              frame True {
                n103 = invoke class="VI" method="FP.Close"(reference=w294, error in=w295) -> (error out=w296:errorcluster)  [unwired: 1 in, 2 out]
              }
            }
          }
          frame "Hidden", "Hide" {
            w297 = T4."Hidden" ("State")
            n104 = property class="VI"(reference=w303, error in=w302) -> (reference out=w300:refnum<vi>, error out=w301:errorcluster, "FP.State"=w299:T4)
            n105 = Not Equal?(x=w299, y=w297) -> (x != y?=w298:bool)
            n106 = case shown="True" w298 {
              tunnel: [w308 w309] -> w304
              tunnel: w301 -> [w307 w309]
              tunnel: w300 -> [w306 _]
              tunnel: w297 -> [w305 _]
              frame True {
                n107 = invoke class="VI" method="FP.Open"(reference=w306, error in=w307, "State"=w305) -> (error out=w308:errorcluster)  [unwired: 2 in, 4 out]
              }
              frame False {
              }
            }
          }
          frame "Minimize", "Minimized" {
            w310 = T4."Minimized" ("State")
            n108 = property class="VI"(reference=w316, error in=w315) -> (reference out=w313:refnum<vi>, error out=w314:errorcluster, "FP.State"=w312:T4)
            n109 = Not Equal?(x=w312, y=w310) -> (x != y?=w311:bool)
            n110 = case shown="True" w311 {
              tunnel: [w321 w322] -> w317
              tunnel: w314 -> [w320 w322]
              tunnel: w313 -> [w319 _]
              tunnel: w310 -> [w318 _]
              frame True {
                n111 = invoke class="VI" method="FP.Open"(reference=w319, error in=w320, "State"=w318) -> (error out=w321:errorcluster)  [unwired: 2 in, 4 out]
              }
              frame False {
              }
            }
          }
          frame "Maximize", "Maximized" {
            w323 = T4."Maximized" ("State")
            n112 = property class="VI"(reference=w329, error in=w328) -> (reference out=w326:refnum<vi>, error out=w327:errorcluster, "FP.State"=w325:T4)
            n113 = Not Equal?(x=w325, y=w323) -> (x != y?=w324:bool)
            n114 = case shown="True" w324 {
              tunnel: [w334 w335] -> w330
              tunnel: w327 -> [w333 w335]
              tunnel: w326 -> [w332 _]
              tunnel: w323 -> [w331 _]
              frame True {
                n115 = invoke class="VI" method="FP.Open"(reference=w332, error in=w333, "State"=w331) -> (error out=w334:errorcluster)  [unwired: 2 in, 4 out]
              }
              frame False {
              }
            }
          }
        }
      }
      frame "---------- Macro ----------" {
        # "Do not put any code in this frame.\n(It is a separator no-op. You can make a copy of this frame to create a new Macro frame)"
        n116 = call <vilib>:"Add State(s) to Queue__JKI_lib_State_Machine.vi"("State(s) in (\"\")"=w340) -> ("States Out"=w339:string)  [unwired: 14 in]
      }
      frame "Macro: Initialize" {
        w342 = "Data: Initialize\nInitialize Core Data\nEvents: Register\nUI: Initialize\nUI: Front Panel State >> Open"  # Data: Initialize Initialize Core Data Events: Register UI: Initialize UI: Front Panel State >> Open
        # "Initialization Macro\n(This is called once, when the VI starts)"
        n117 = call <vilib>:"Add State(s) to Queue__JKI_lib_State_Machine.vi"("State(s) in Front (\"\")"=w342, "State(s) in (\"\")"=w346) -> ("States Out"=w345:string)  [unwired: 13 in]
      }
      frame "Macro: Exit" {
        # "#CSM-Example Step5"
        # "Exit Macro\n(This is called once, when the VI exits)"
        n118 = Unbundle By Name(w356) -> ("Core.Close Panel on Exit?"=w355:bool)
        n119 = Select(t="UI: Front Panel State >> Close", s=w355, f="") -> (s? t:f=w352:string)
        n120 = call "CSM - Build Exit Messages of CSMs.vi"("CSMs"=string[] ["Worker"]) -> ("States"=w347:string)  [unwired: 14 in]
        n121 = call <vilib>:"Add State(s) to Queue__JKI_lib_State_Machine.vi"("State(s) in Front (\"\")"=w347, "State(s) in (\"\")"=w352, "State(s) at Back (\"\")"="Data: Cleanup\nEvents: Unregister\nExit") -> ("States Out"=w350:string)  [unwired: 12 in]
        n122 = call <vilib>:"Add State(s) to Queue__JKI_lib_State_Machine.vi"("State(s) in Front (\"\")"=w350, "State(s) in (\"\")"=w359) -> ("States Out"=w358:string)  [unwired: 13 in]
      }
    }
  }
  n123 = while {
    tunnel: w1 -> [w362]
    stop <- w363 stop-if-true
    n124 = call "CSM - Module Turns Invalid.vi"("CSM Name"=w362) -> ("Turn Invalid (Exit)?"=w363:bool)  [unwired: 2 in]
    n125 = call "CSM - List Modules.vi"("With Nodes? (F)"="All?") -> ("Module Names"=w364:string[])  [unwired: 9 in, 1 out]
    n126 = for {
      tunnel: w364 -> [w372] mode=indexing
      tunnel: [w367] -> w365 mode=indexing
      n127 = call "CSM - Module Status.vi"("CSM Name"=w372) -> ("error out"=w366:errorcluster, "#Nodes"=w369:i32, "Mode"=w370:T1, "CSM Name (Dup)"=w371:string, "#Elements In Queue"=w368:i32)  [unwired: 6 in]
      n128 = Bundle("CSM Name (Dup)"=w371, "Mode"=w370, "#Nodes"=w369, "#Elements In Queue"=w368) -> (w367:T8)  [unwired: 1 in]
      n129 = call <vilib>:"Clear Errors.vi"("error in (no error)"=w366) -> ()  [unwired: 5 in, 2 out]
    }
    "Module List" <- w365
    n130 = Wait (ms)(milliseconds to wait=u32 100) -> ()  [unwired: 1 out]
  }
